vi "StartStop.vi"(8 "error in (no error)":errorcluster, 10 "StartStop":bool, 11 "Generador de funciones in":refnum<class "Generador de funciones.lvclass">) -> (0 "error out":errorcluster, 3 "Generador de funciones out":refnum<class "Generador de funciones.lvclass">)   [LabVIEW 2019, in "Generador de funciones.lvlib" / "Generador de funciones.lvclass"]
uses:
  Generador de funciones.lvclass
  Generador de funciones.lvclass/Generador de funciones.ctl
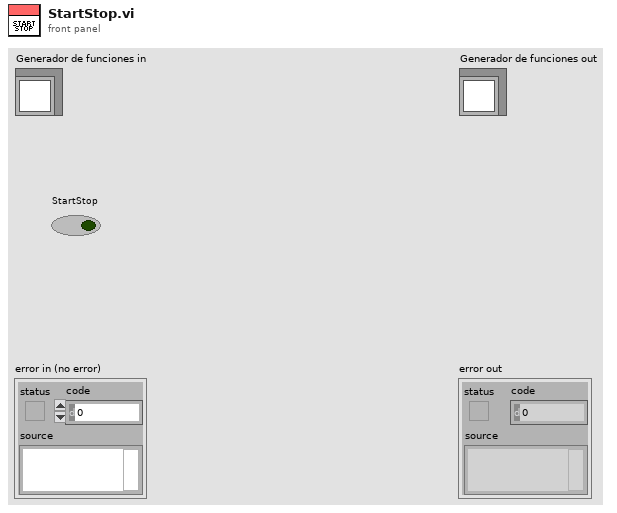
[diagram p1: front panel]
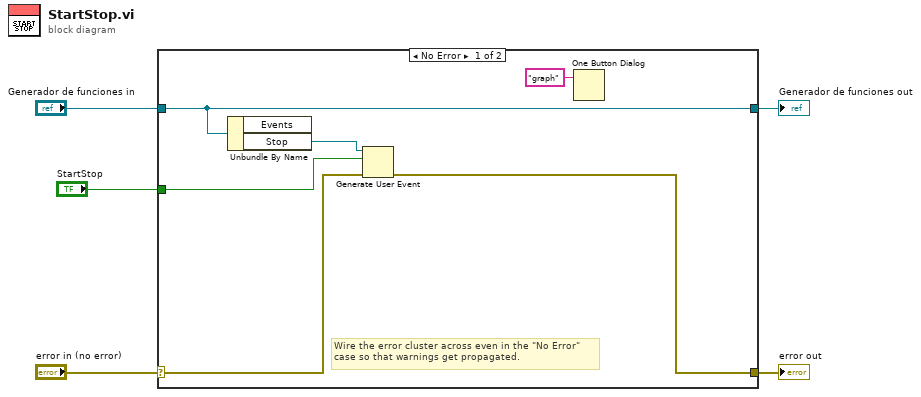
[diagram p0: block diagram]
diagram:
  n1 = case shown="No Error" "error in (no error)" {
    selector: "error in (no error)" -> [w8 w13]
    tunnel: [w7 w13] -> w4
    tunnel: [w11 w12] -> w2
    tunnel: "Generador de funciones in" -> [w11 w12]
    tunnel: "StartStop" -> [w9 _]
    frame No Error {
      # "Wire the error cluster across even in the \"No Error\"\ncase so that warnings get propagated."
      n2 = Unbundle By Name(w11) -> ("Stop"=w10:refnum<user-event>)  [unwired: 1 out]
      n3 = Generate User Event(user event=w10, event data cluster=w9, error in=w8) -> (error out=w7:errorcluster)  [unwired: 1 in, 1 out]
      n4 = One Button Dialog(message="graph") -> ()  [unwired: 1 in, 1 out]
    }
    frame Error {
    }
  }
  "error out" <- w4
  "Generador de funciones out" <- w2
